vi "ClimbLogic.vi"(0 "Climb":dbl, 5 "ClimbDriveAxis":dbl, 7 "ClimbIRVal":dbl, 9 "UpFront":bool, 11 "UpBack":bool, 12 "AutomaticClimb":bool) -> (4 "ActuateFrontClimb":dbl, 6 "ActuateBackClimb":dbl, 10 "ClimbDrive":dbl)   [LabVIEW 2018]
uses:
  Swerve/SwerveGlobals.vi
  <vilib>/Rock Robotics/WPI/Utilities/WPI_GetSetVariantRefNum.vi
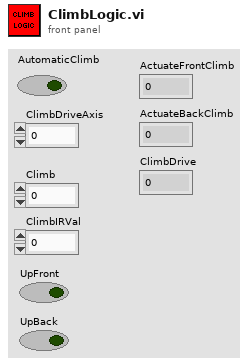
[diagram p1: front panel]
types:
  T1 = typedef "WPI_CompressorDevRef.ctl" = cluster{"DevStatus":errorcluster, "Pneumatics Control Module":u8}
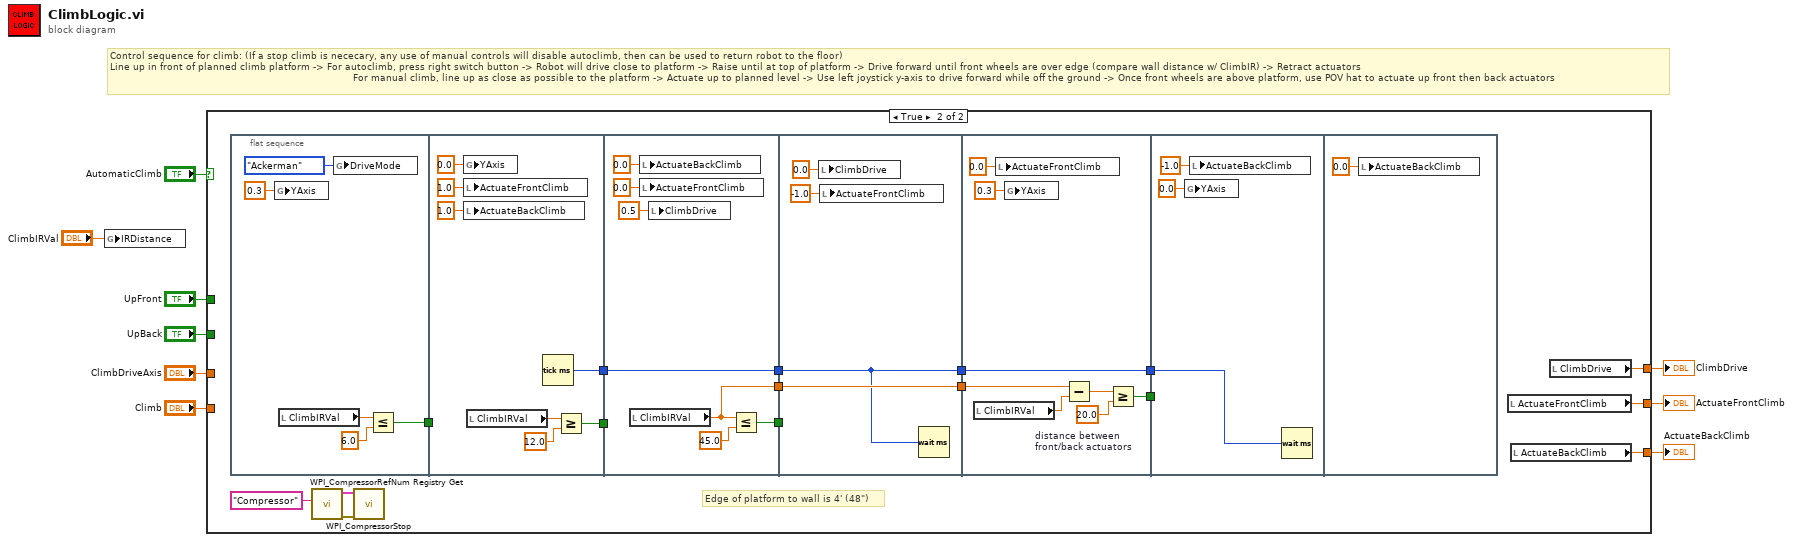
[diagram p0: block diagram]
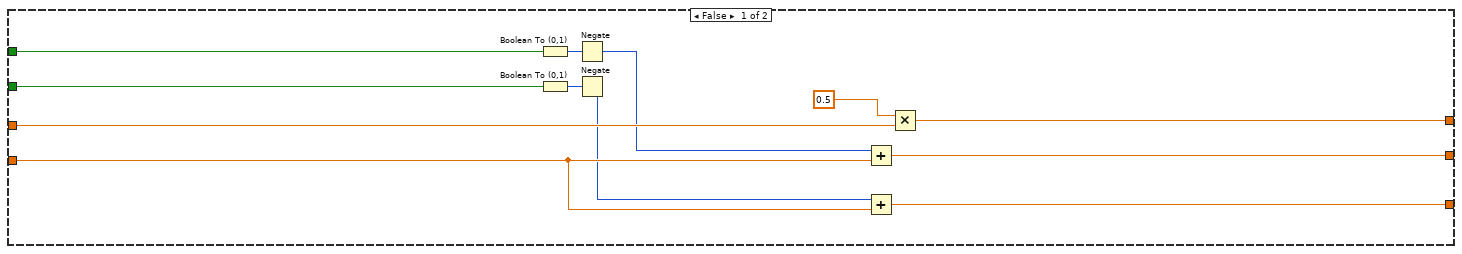
[diagram p2: hidden frame]
diagram:
  # "Control sequence for climb: (If a stop climb is nececary, any use of manual controls will disable autoclimb, then can be used to return robot to the floor)\nLine up in front of planned climb platform -> For autoclimb, press right switch button -> Robot will drive close to platform -> Raise until at top of platform -> Drive forward until front wheels are over edge (compare wall distance w/ ClimbIR) -> Retract actuators\n                                                                                 For manual climb, line up as close as possible to the platform -> Actuate up to planned level -> Use left joystick y-axis to drive forward while off the ground -> Once front wheels are above platform, use POV hat to actuate up front then back actuators"
  n1 = global write "SwerveGlobals.vi" "IRDistance"("ClimbIRVal") -> ()
  n2 = case shown="True" "AutomaticClimb" {
    tunnel: [w20 w26] -> w6
    tunnel: "Climb" -> [w13 _]
    tunnel: [w11 w27] -> w5
    tunnel: "ClimbDriveAxis" -> [w21 _]
    tunnel: [w14 w25] -> w4
    tunnel: "UpFront" -> [w19 _]
    tunnel: "UpBack" -> [w15 _]
    frame False {
      n3 = Boolean To (0,1)(Boolean=w19) -> (0, 1=w18:i16)
      n4 = Boolean To (0,1)(Boolean=w15) -> (0, 1=w16:i16)
      n5 = Negate(x=w18) -> (-x=w17:i16)
      n6 = Negate(x=w16) -> (-x=w12:i16)
      n7 = Add(x=w17, y=w13) -> (x+y=w20:dbl)
      n8 = Add(x=w12, y=w13) -> (x+y=w14:dbl)
      n9 = Multiply(x=0.5, y=w21) -> (x*y=w11:dbl)
    }
    frame True {
      # "Edge of platform to wall is 4' (48\")"
      n10 = flat-sequence {
        tunnel: [w38] -> w37
        tunnel: w37 -> [_]
        tunnel: [w44] -> w36
        tunnel: [w43] -> w33
        tunnel: w36 -> [_]
        tunnel: [w53] -> w35
        tunnel: [w51] -> w34
        tunnel: w33 -> [w51]
        tunnel: [w50] -> w32
        tunnel: w35 -> [_]
        tunnel: w34 -> [w57]
        tunnel: w32 -> [w58]
        tunnel: [w58] -> w31
        tunnel: [w57] -> w28
        tunnel: w31 -> [w65]
        tunnel: [w62] -> w30
        tunnel: [w61] -> w29
        tunnel: w28 -> [w61]
        tunnel: w30 -> [_]
        tunnel: w29 -> [w69]
        frame #0 {
          n11 = global write "SwerveGlobals.vi" "YAxis"(0.3 ("YAxis")) -> ()
          n12 = local read "ClimbIRVal"() -> (w40:dbl)
          n13 = global write "SwerveGlobals.vi" "DriveMode"(enum16{"Swerve", "Ackerman"}."Ackerman" ("DriveMode")) -> ()
          n14 = Less Or Equal?(x=w40, y=6.0) -> (x <= y?=w38:bool)
        }
        frame #1 {
          n15 = global write "SwerveGlobals.vi" "YAxis"(0.0 ("YAxis")) -> ()
          n16 = local write "ActuateFrontClimb"(1.0 ("ActuateFrontClimb")) -> ()
          n17 = local write "ActuateBackClimb"(1.0 ("ActuateBackClimb")) -> ()
          n18 = local read "ClimbIRVal"() -> (w46:dbl)
          n19 = Tick Count (ms)() -> (millisecond timer value=w43:u32)
          n20 = Greater Or Equal?(x=w46, y=12.0) -> (x >= y?=w44:bool)
        }
        frame #2 {
          n21 = local read "ClimbIRVal"() -> (w50:dbl)
          n22 = local write "ActuateBackClimb"(0.0 ("ActuateBackClimb")) -> ()
          n23 = local write "ActuateFrontClimb"(0.0 ("ActuateFrontClimb")) -> ()
          n24 = local write "ClimbDrive"(0.5 ("ClimbDrive")) -> ()
          n25 = Less Or Equal?(x=w50, y=45.0) -> (x <= y?=w53:bool)
        }
        frame #3 {
          n26 = local write "ClimbDrive"(0.0 ("ClimbDrive")) -> ()
          n27 = local write "ActuateFrontClimb"(-1.0 ("ActuateFrontClimb")) -> ()
          n28 = Wait (ms)(milliseconds to wait=w57) -> ()  [unwired: 1 out]
        }
        frame #4 {
          w66 = 20.0  # distance between front/back actuators
          n29 = local read "ClimbIRVal"() -> (w64:dbl)
          n30 = local write "ActuateFrontClimb"(0.0 ("ActuateFrontClimb")) -> ()
          n31 = global write "SwerveGlobals.vi" "YAxis"(0.3 ("YAxis")) -> ()
          n32 = Subtract(x=w65, y=w64) -> (x-y=w63:dbl)
          n33 = Greater Or Equal?(x=w63, y=w66) -> (x >= y?=w62:bool)
        }
        frame #5 {
          n34 = global write "SwerveGlobals.vi" "YAxis"(0.0 ("YAxis")) -> ()
          n35 = local write "ActuateBackClimb"(-1.0 ("ActuateBackClimb")) -> ()
          n36 = Wait (ms)(milliseconds to wait=w69) -> ()  [unwired: 1 out]
        }
        frame #6 {
          n37 = local write "ActuateBackClimb"(0.0 ("ActuateBackClimb")) -> ()
        }
      }
      n38 = call <vilib>:"WPI_CompressorRefNum Registry Get.vi"("refnum name"="Compressor") -> ("error out"=w23:errorcluster, "CompressorDevRef"=w24:T1)  [unwired: 9 in]
      n39 = call <vilib>:"WPI_CompressorStop.vi"("error in (no error)"=w23, "CompressorDevRef"=w24) -> ()  [unwired: 8 in, 2 out]
      n40 = local read "ActuateFrontClimb"() -> (w26:dbl)
      n41 = local read "ActuateBackClimb"() -> (w25:dbl)
      n42 = local read "ClimbDrive"() -> (w27:dbl)
    }
  }
  "ActuateFrontClimb" <- w6
  "ClimbDrive" <- w5
  "ActuateBackClimb" <- w4
